vi "Stop Core.vi"(10 "final error code":i32, 11 "object in":refnum<class "TableLogger_Actor.lvclass">) -> (3 "object out":refnum<class "TableLogger_Actor.lvclass">)   [LabVIEW 2014, in "TableLogger_Actor.lvlib" / "TableLogger_Actor.lvclass"]
uses:
  TableLogger_Actor.lvclass
  <vilib>/ActorFramework/Actor/Actor.lvclass
panel:
  # "Connector Pane"
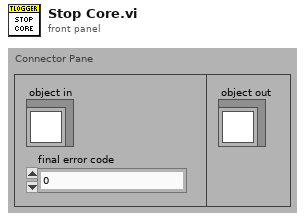
[diagram p1: front panel]
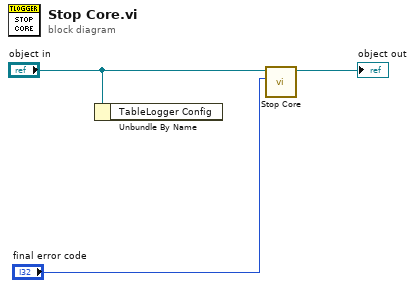
[diagram p0: block diagram]
diagram:
  n1 = Unbundle By Name("object in") -> ()  [unwired: 1 out]
  n2 = call-parent "Stop Core.vi"("final error code"="final error code", "Actor in"="object in") -> ("Actor out"=→"object out":refnum<class "TableLogger_Actor.lvclass">)  [unwired: 9 in]
